vi "切换时钟开关.vi"(8 "error in":errorcluster caption="error constant", 9 "OUT":u16, 11 "IN":u16) -> (0 "error out":errorcluster caption="error constant", 1 "ask":string, 2 "Isfailed":bool)   [LabVIEW 2015]
uses:
  Global/SeverGlobal.vi
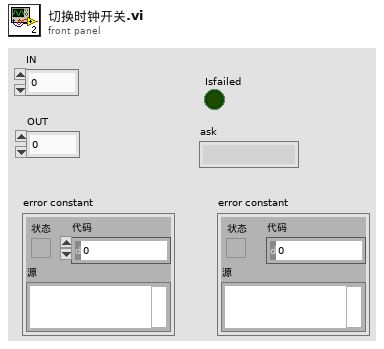
[diagram p1: front panel]
types:
  T1 = cluster{"IP_A":string, "PORT_A":i32, "IP_B":string, "PORT_B":i32, "IP_CLK":string, "PORT_CLK":i32, "IP_SWITCH":string, "PORT_SWITCH":i32}
  T2 = enum16{"Standard", "Buffered", "CRLF", "Immediate"}
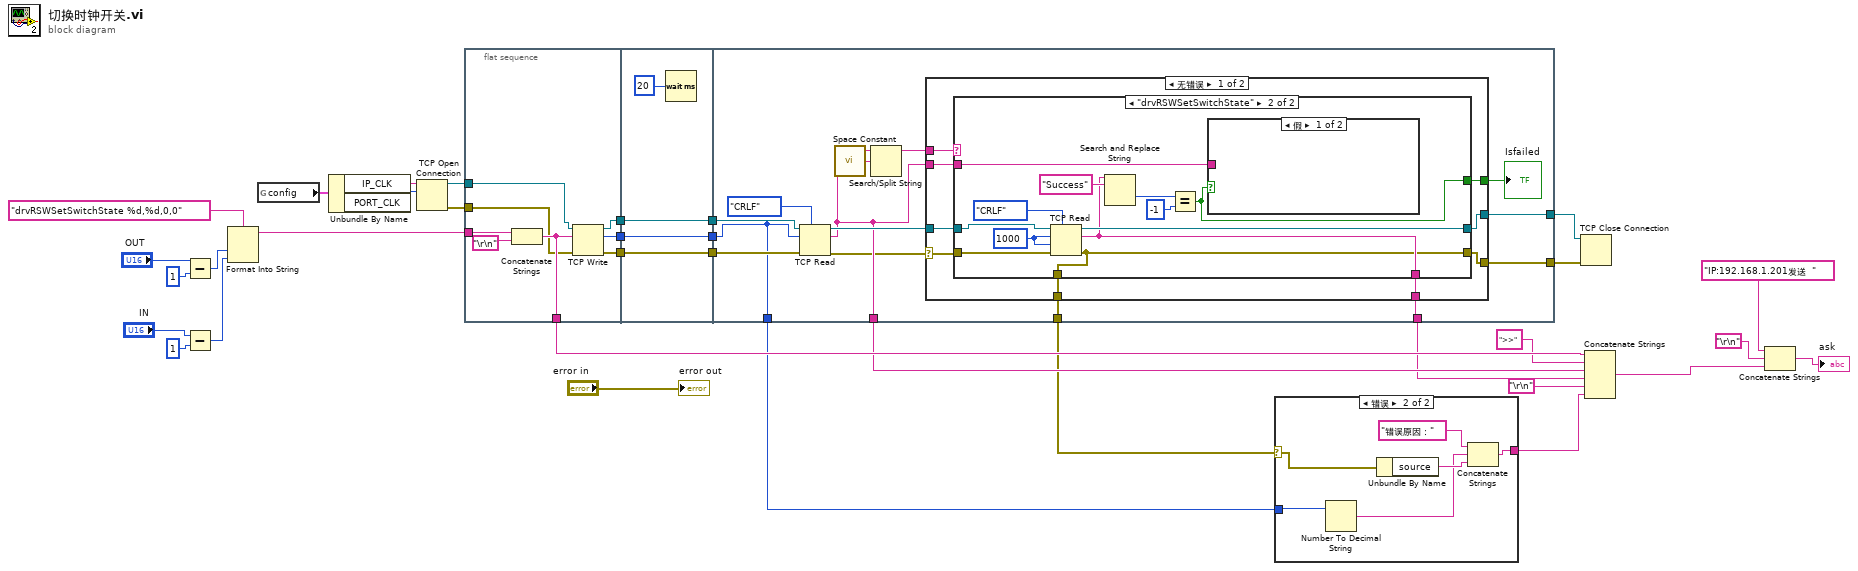
[diagram p0: block diagram]
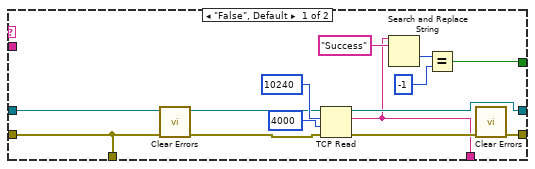
[diagram p3: hidden frame]
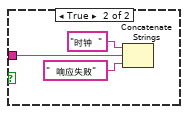
[diagram p4: hidden frame]
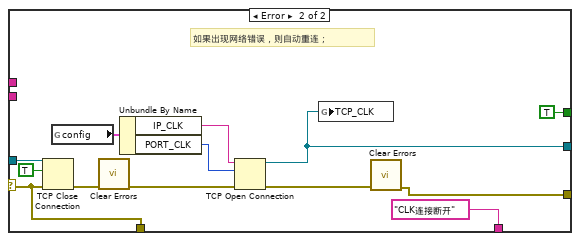
[diagram p5: hidden frame]
diagram:
  n1 = Subtract(x="OUT", y=1) -> (x-y=w32:i32)
  n2 = Subtract(x="IN", y=1) -> (x-y=w30:i32)
  n3 = Format Into String(format string="drvRSWSetSwitchState %d,%d,0,0" ("格式字符串"), w32, w30) -> (resulting string=w29:string)  [unwired: 2 in, 1 out]
  n4 = global read "SeverGlobal.vi" "config"() -> (w7:T1)
  n5 = Unbundle By Name(w7) -> ("IP_CLK"=w6:string, "PORT_CLK"=w5:i32)
  n6 = TCP Open Connection(address=w6, remote port or service name=w5) -> (connection ID=w4:refnum<k5>, error out=w3:errorcluster)  [unwired: 3 in]
  n7 = flat-sequence {
    tunnel: [w40] -> w27
    tunnel: [w39] -> w25
    tunnel: [w38] -> w23
    tunnel: [w37] -> w16
    tunnel: w29 -> [w41]
    tunnel: w4 -> [w36]
    tunnel: w3 -> [w35]
    tunnel: [w45] -> w28
    tunnel: w27 -> [w45]
    tunnel: [w44] -> w26
    tunnel: w25 -> [w44]
    tunnel: [w43] -> w24
    tunnel: w23 -> [w43]
    tunnel: w28 -> [w56]
    tunnel: w26 -> [w49]
    tunnel: w24 -> [w55]
    tunnel: [w53] -> w14
    tunnel: [w52] -> w13
    tunnel: [w51] -> w11
    tunnel: [w49] -> w8
    tunnel: [w48] -> w2
    tunnel: [w47] -> w1
    frame #0 {
      n8 = Concatenate Strings(w41, "\r\n") -> (w37:string)
      n9 = TCP Write(connection ID=w36, data in=w37, error in (no error)=w35) -> (connection ID out=w40:refnum<k5>, bytes written=w39:i32, error out=w38:errorcluster)  [unwired: 1 in]
    }
    frame #1 {
      n10 = Wait (ms)(milliseconds to wait=u32 20 ("delay")) -> ()  [unwired: 1 out]
    }
    frame #2 {
      n11 = TCP Read(connection ID=w56, bytes to read=w49, error in (no error)=w55, 7:T2."CRLF" ("mode (standard)")) -> (connection ID out=w57:refnum<k5>, data out=w53:string, error out=w50:errorcluster)  [unwired: 1 in]
      n12 = call <vilib>:"Space Constant.vi"() -> ("String"=w60:string)
      n13 = Search/Split String(string=w53, search string/char (-)=w60) -> (substring before match=w58:string)  [unwired: 1 in, 2 out]
      n14 = case shown="无错误" w50 {
        selector: w50 -> [w63 w101]
        tunnel: w58 -> [w69 _]
        tunnel: w57 -> [w68 w104]
        tunnel: [w67 TRUE] -> w54
        tunnel: w53 -> [w66 _]
        tunnel: [w65 "CLK连接断开" ("字符串")] -> w52
        tunnel: [w64 w101] -> w51
        tunnel: [w61 w99] -> w48
        tunnel: [w62 w98] -> w47
        frame No Error {
          n15 = case shown="\"drvRSWSetSwitchState\"" w69 {
            tunnel: [w78 w93] -> w62
            tunnel: [w77 w83] -> w61
            tunnel: w68 -> [w79 w92]
            tunnel: w63 -> [w70 w91]
            tunnel: w66 -> [_ w86]
            tunnel: [w72 w85] -> w67
            tunnel: [w73 w84] -> w65
            tunnel: [w70 w83] -> w64
            frame "False", Default {
              n16 = call <vilib>:"Clear Errors.vi"("error in (no error)"=w70) -> ("error out"=w71:errorcluster)  [unwired: 5 in, 1 out]
              n17 = TCP Read(connection ID=w79, bytes to read=10240, error in (no error)=w71, 9:4000 ("timeout ms (25000)")) -> (connection ID out=w78:refnum<k5>, data out=w73:string, error out=w81:errorcluster)  [unwired: 1 in]
              n18 = Search and Replace String(input string=w73, search string="Success") -> (offset past replacement=w74:i32)  [unwired: 6 in, 3 out]
              n19 = Equal?(x=w74, y=-1) -> (x = y?=w72:bool)
              n20 = call <vilib>:"Clear Errors.vi"("error in (no error)"=w81) -> ("error out"=w77:errorcluster)  [unwired: 5 in, 1 out]
            }
            frame "drvRSWSetSwitchState" {
              w90 = 1000 ("timeout ms (25000)")
              n21 = TCP Read(connection ID=w92, bytes to read=w90, error in (no error)=w91, 7:T2."CRLF" ("mode (standard)"), 9:w90) -> (connection ID out=w93:refnum<k5>, data out=w84:string, error out=w83:errorcluster)
              n22 = Search and Replace String(input string=w84, search string="Success") -> (offset past replacement=w88:i32)  [unwired: 6 in, 3 out]
              n23 = Equal?(x=w88, y=-1) -> (x = y?=w85:bool)
              n24 = case shown="假" w85 {
                tunnel: w86 -> [_ w97]
                frame False {
                }
                frame True {
                  n25 = Concatenate Strings("时钟  " ("message"), w97, "  响应失败" ("message")) -> ()  [unwired: 1 out]
                }
              }
            }
          }
        }
        frame Error {
          # "如果出现网络错误，则自动重连；"
          n26 = TCP Close Connection(connection ID=w104, abort (F)=TRUE ("中止(F)"), error in (no error)=w101) -> (error out=w105:errorcluster)  [unwired: 1 out]
          n27 = global read "SeverGlobal.vi" "config"() -> (w107:T1)
          n28 = call <vilib>:"Clear Errors.vi"("error in (no error)"=w105) -> ("error out"=w106:errorcluster)  [unwired: 5 in, 1 out]
          n29 = Unbundle By Name(w107) -> ("IP_CLK"=w108:string, "PORT_CLK"=w109:i32)
          n30 = TCP Open Connection(address=w108, remote port or service name=w109, error in (no error)=w106) -> (connection ID=w98:refnum<k5>, error out=w110:errorcluster)  [unwired: 2 in]
          n31 = global write "SeverGlobal.vi" "TCP_CLK"(w98) -> ()
          n32 = call <vilib>:"Clear Errors.vi"("error in (no error)"=w110) -> ("error out"=w99:errorcluster)  [unwired: 5 in, 1 out]
        }
      }
      "Isfailed" <- w54
    }
  }
  n33 = case shown="错误" w11 {
    selector: w11 -> [_ w116]
    tunnel: [_ w114] -> w9
    tunnel: w8 -> [_ w112]
    frame No Error {
    }
    frame Error {
      n34 = Number To Decimal String(number=w112) -> (decimal integer string=w111:string)  [unwired: 1 in]
      n35 = Unbundle By Name(w116) -> ("source"=w113:string)
      n36 = Concatenate Strings("错误原因：", w111, w113) -> (w114:string)
    }
  }
  n37 = TCP Close Connection(connection ID=w1, error in (no error)=w2) -> ()  [unwired: 1 in, 2 out]
  n38 = Concatenate Strings(w16, ">>" ("字符串"), w14, w13, "\r\n", w9) -> (w12:string)
  n39 = Concatenate Strings("IP:192.168.1.201发送  " ("delimiter (Tab)"), "\r\n", w12) -> (→"ask":string)
  "error out" <- "error in"
